vi "Write Separate UI.vi"(8 "error in (no error)":errorcluster, 10 "Separate UI":bool, 11 "Mag Lab Root in":refnum<class "Mag Lab Root.lvclass">) -> (0 "error out":errorcluster, 3 "Mag Lab Root out":refnum<class "Mag Lab Root.lvclass">)   [LabVIEW 2015, in "Mag Lab Root.lvclass"]
uses:
  Mag Lab Root.lvclass
  Mag Lab Root.lvclass/Mag Lab Root.ctl
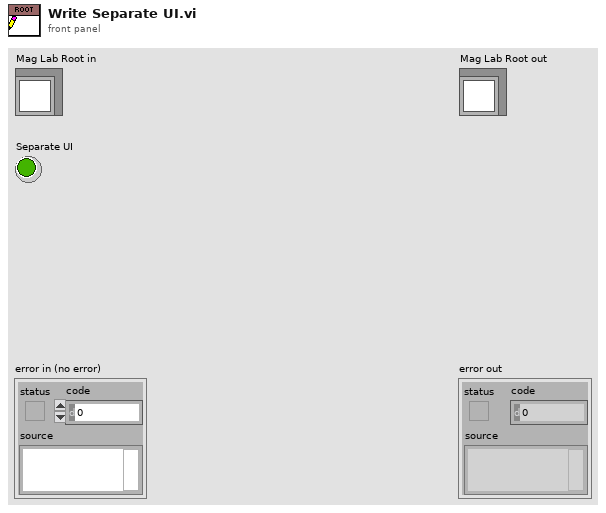
[diagram p1: front panel]
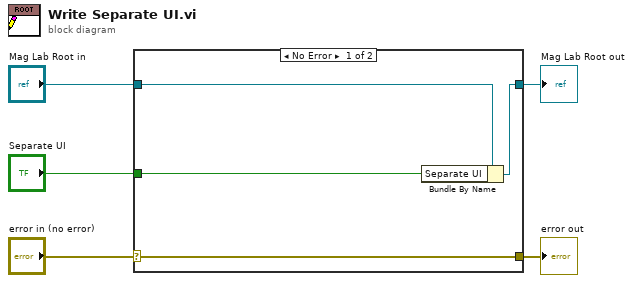
[diagram p0: block diagram]
diagram:
  n1 = case shown="No Error" "error in (no error)" {
    selector: "error in (no error)" -> [w9 w10]
    tunnel: [w9 w10] -> w4
    tunnel: [w7 w11] -> w2
    tunnel: "Mag Lab Root in" -> [w8 w11]
    tunnel: "Separate UI" -> [w6 _]
    frame No Error {
      n2 = Bundle By Name(cluster=w8, "Separate UI"=w6) -> (w7:refnum<class "Mag Lab Root.lvclass">)
    }
    frame Error {
    }
  }
  "error out" <- w4
  "Mag Lab Root out" <- w2
